vi "mainVI.vi"() -> ()   [LabVIEW 2013]
panel:
  out "Waveform Graph":dbl[](graph)
  out "stringa":string
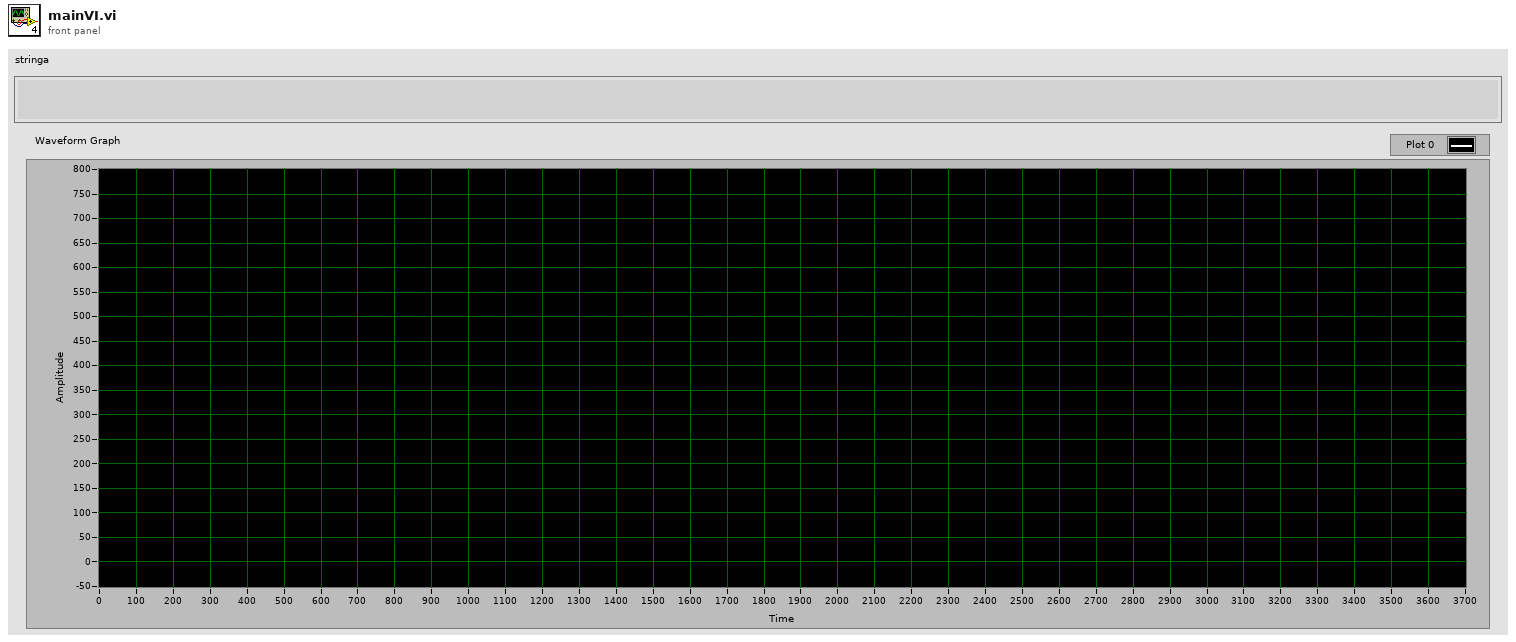
[diagram p1: front panel]
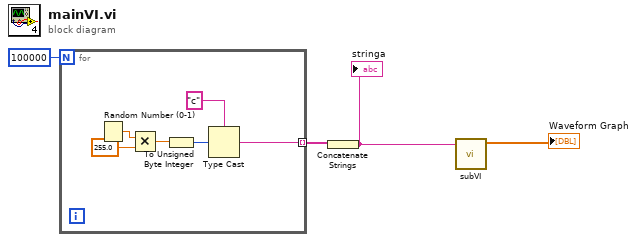
[diagram p0: block diagram]
diagram:
  n1 = for {
    N: 100000 -> [_]
    tunnel: [w5] -> w3 mode=indexing
    n2 = Random Number (0-1)() -> (number: 0 to 1=w10:dbl)
    n3 = Multiply(x=w10, y=255.0) -> (x*y=w8:dbl)
    n4 = To Unsigned Byte Integer(number=w8) -> (unsigned 8bit integer=w7:u8)
    n5 = Type Cast(type="c", x=w7) -> (*(type *) &x=w5:string)
  }
  n6 = Concatenate Strings(w3) -> (w2:string)
  "stringa" <- w2
  n7 = call "subVI.vi"("String"=w2) -> ("numeri"=→"Waveform Graph":dbl[])  [unwired: 10 in]
